vi "RRTPlan.vi"(8 "Initial Pos x,y":dbl[](array[numeric]), 9 "Dest x,y":dbl[](array[numeric]), 10 "IA State":T3={"our_robots"=[], "enemy_robots"=[], "balls"=[], "geometry"={"line_width"=0, "field_length"=0, "field_width"=0, "boundary_width"=0, "referee_width"=0, "goal_width"=0, "goal_depth"=0, "goal_wall_width"=0, "center_circle_radius"=0, "defense_radius"=0, "defense_stretch"=0, "free_kick_from_defense_dist"=0, "penalty_spot_from_field_line_dist"=0, "penalty_line_from_spot_dist"=0}, "IA Judge"={"stage"="", "command"="", "our_goalie_id"=0.0, "enemy_goalie_id"=0.0, "command enum"=enum."Halt", "Time"=enum."Azul"}, "Received Timestamp"=timestamp(0 s since 1904-01-01), "Events"={"Touch"=FALSE, "Ball out"=FALSE, "id touch"=0.0, "Ball out of \nVision"=FALSE, "Ball inside \nGoalie area"=FALSE, "Robot not responding"=FALSE, "Robots responding status"=[1.0, 1.0, 1.0, 1.0, 1.0, 1.0], "Enemy Ball \nPossession"=FALSE, "Pass State"=FALSE, "id end of pass"=0.0, "Kick"=FALSE, "Id ini Possession"=0.0, "Ball Possesion"=FALSE, "Id Possesion"=0.0}}, 11 "Robot":T4={"id"=0, "function"=enum."Attacker", "x"=0.0, "y"=0.0, "orientation"=0.0, "v_tangent"=0.0, "v_normal"=0.0, "v_ang"=0.0, "kick_x"=0.0, "kick_z"=0.0, "dribble"=FALSE, "Timestamp"=timestamp(0 s since 1904-01-01), "estimatives"={"est_v_tangent"=0.0, "est_v_normal"=0.0, "est_vx"=0.0, "est_vy"=0.0, "Pos Robot Est"=[]}, "dest_x_kick"=0.0, "dest_y_kick"=0.0, "Gap Coord"=[], "States"=enum."GoToTangent", "Path "=[], "Path  Smooth"=[], "Dest"=[]}) -> (0 "Path":dbl[][](array[numeric]), 1 "Smooth Path":dbl[][](array[numeric]))   [LabVIEW 2017]
uses:
  Core/AI Robot.ctl
  Intel/Functions Enum.ctl
  Intel/AttackerStates.ctl
  PathDests.ctl
  PathDest.ctl
  Core/AI Input.ctl
  Core/AI Ball.ctl
  Core/Field Size.ctl
  Core/AI Judge.ctl
  Intel/Command Enum.ctl
  Util/Events/Events.ctl
  kD-tree/KD-Tree.ctl
  kD-tree/Node.ctl
  <vilib>/Analysis/_algsub.llb/Real Vector Norm.vi
  <vilib>/Analysis/NI_AALPro.lvlib
panel:
  out "New KD-Tree":T1
  out "x > y? 2":bool
  out "Modulo":dbl
  in  "WayPointProb":dbl=0.6 format="%#_13g"
  in  "GoalProb":dbl=0.1 format="%#_13g"
  in  "Step":dbl=80.0
  out "Elapsed Time (s)":dbl
  out "Time has Elapsed":bool
  in  "threshold":dbl=80.0
  out "Goal":dbl[](array[numeric])
  out "Initial State":dbl[](array[numeric])
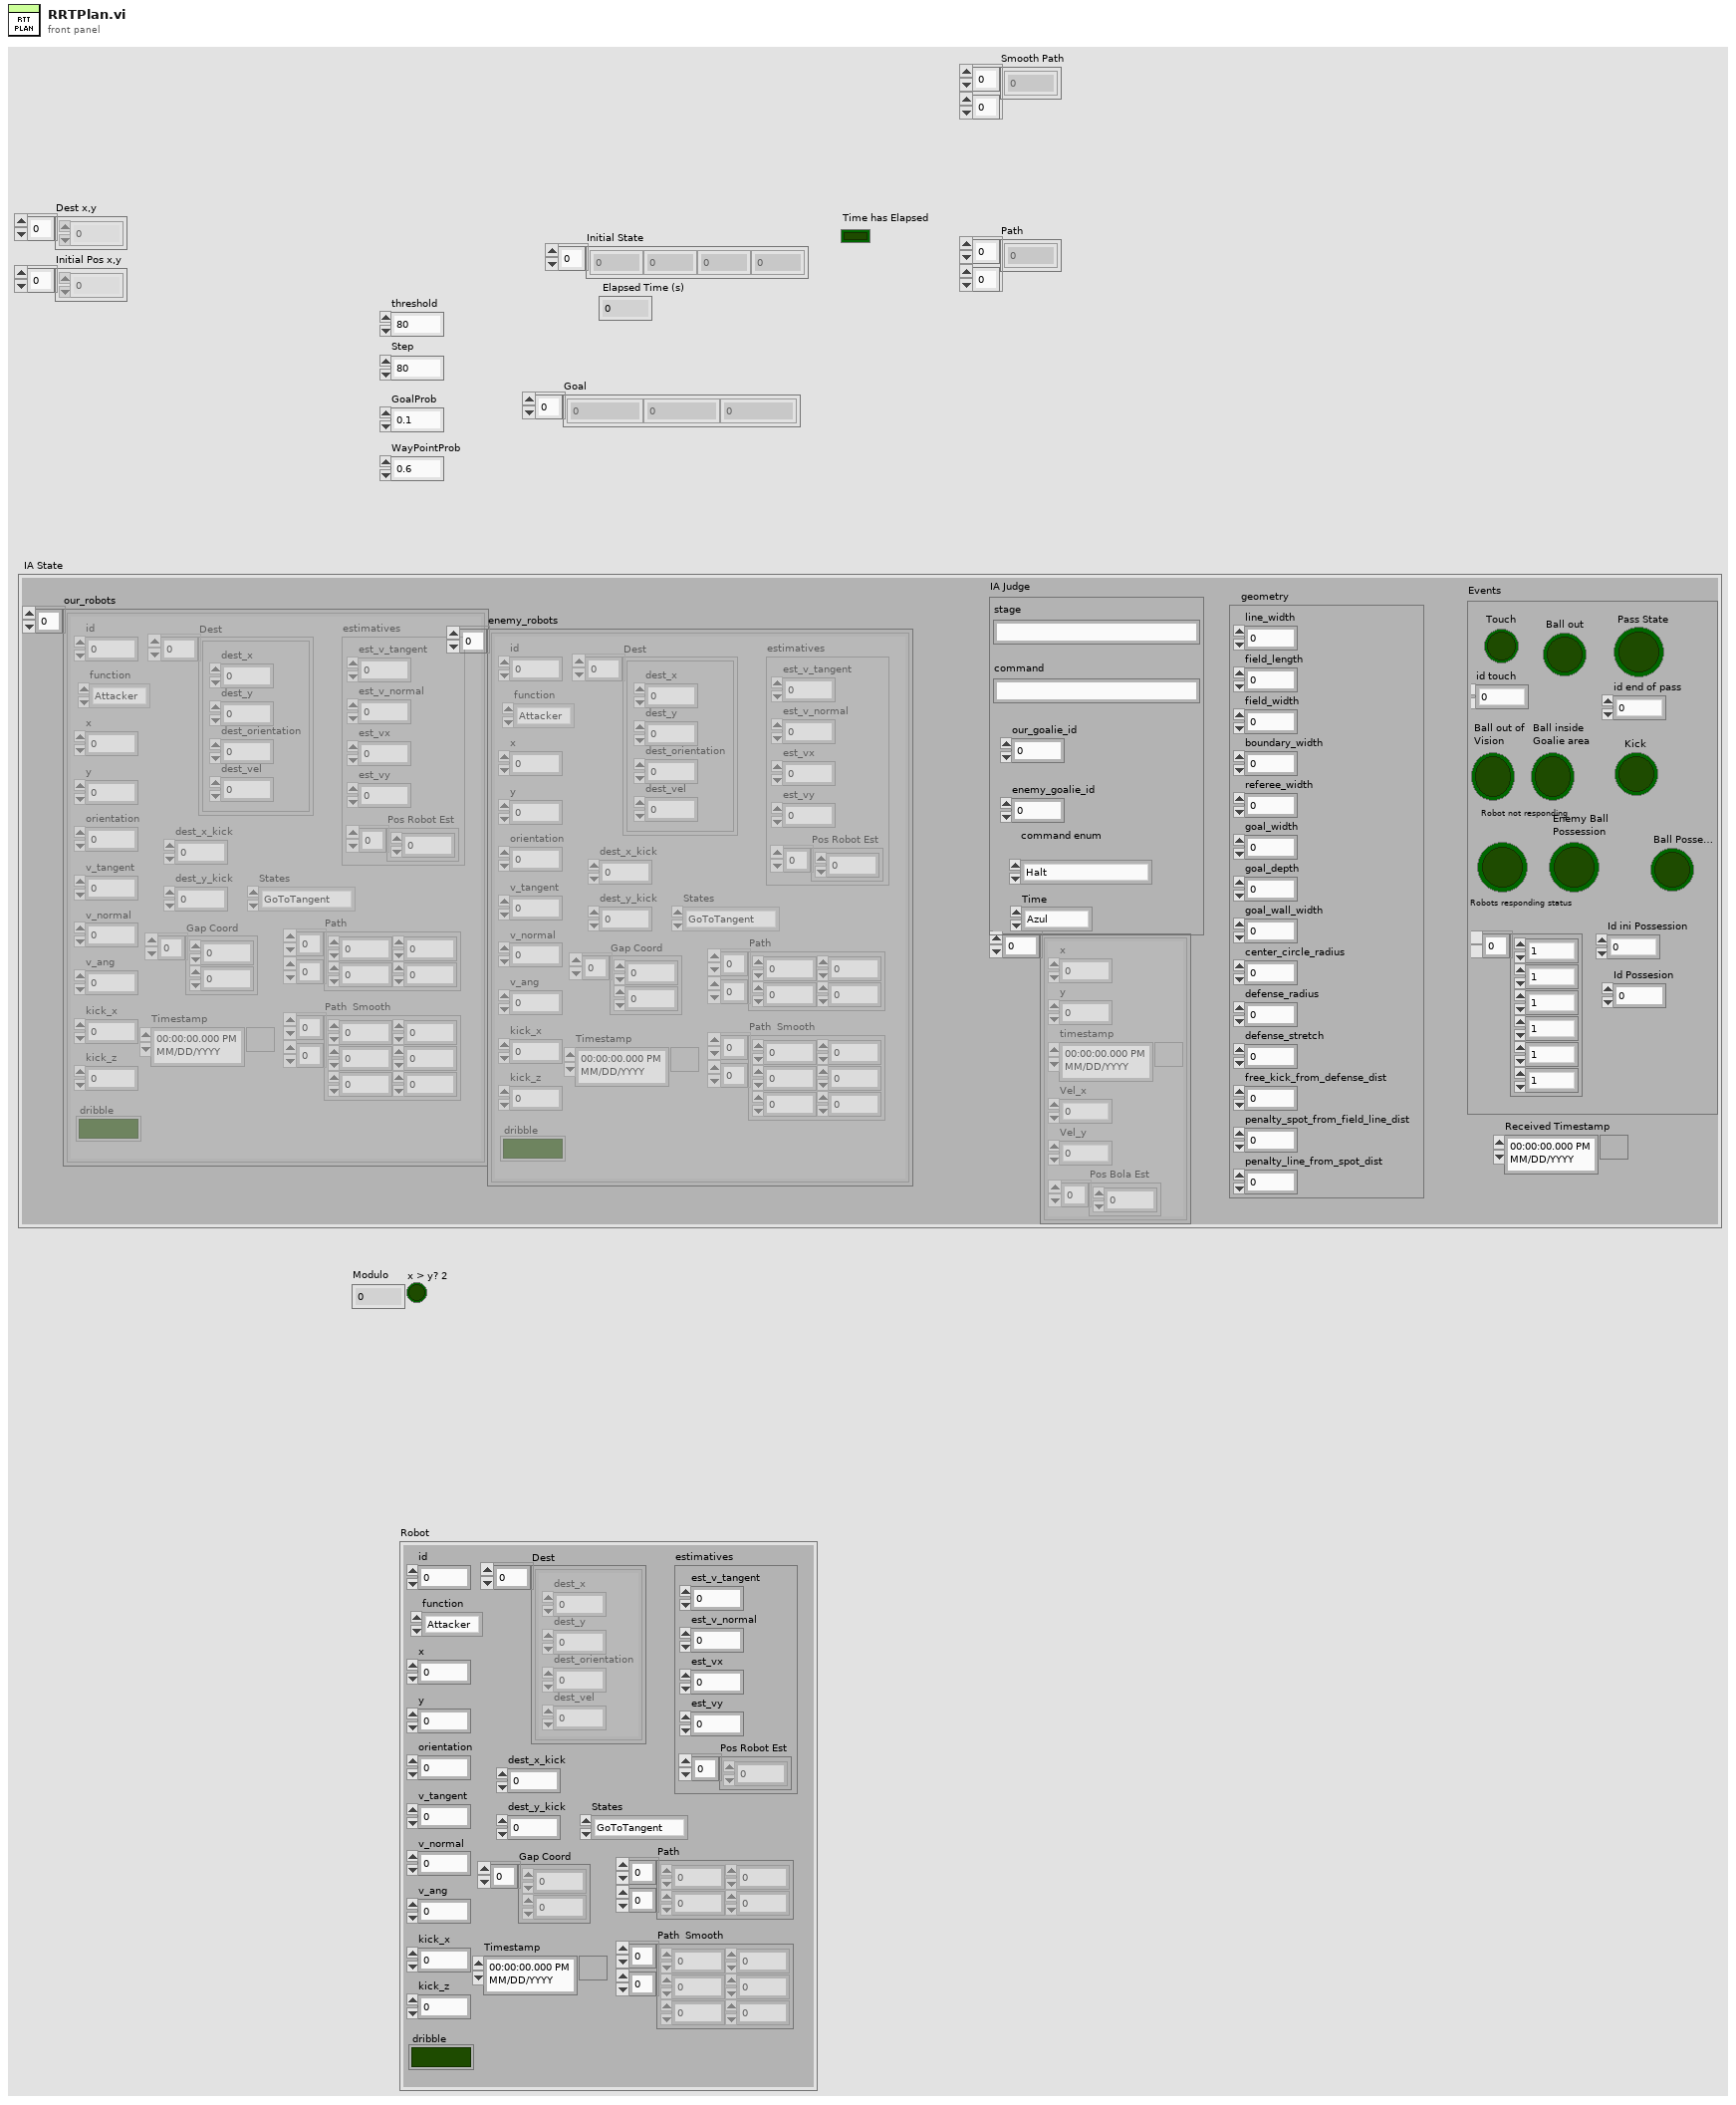
[diagram p1: front panel]
types:
  T1 = typedef "KD-Tree.ctl" = T2[]
  T2 = typedef "Node.ctl" = cluster{"axis":enum16{"null", "x", "y"}, "value":dbl, "left":dbl, "right":dbl, "Point":dbl[]}
  T3 = typedef "AI Input.ctl" = cluster{"our_robots":T4[], "enemy_robots":T4[], "balls":T9[], "geometry":T10, "IA Judge":T11, "Received Timestamp":timestamp, "Events":T13}
  T4 = typedef "AI Robot.ctl" = cluster{"id":u32, "function":T5, "x":dbl, "y":dbl, "orientation":dbl, "v_tangent":dbl, "v_normal":dbl, "v_ang":dbl, "kick_x":dbl, "kick_z":dbl, "dribble":bool, "Timestamp":timestamp, "estimatives":cluster{"est_v_tangent":dbl, "est_v_normal":dbl, "est_vx":dbl, "est_vy":dbl, "Pos Robot Est":dbl[]}, "dest_x_kick":dbl, "dest_y_kick":dbl, "Gap Coord":dbl[], "States":T6, "Path ":dbl[][], "Path  Smooth":dbl[][], "Dest":T7}
  T5 = typedef "Functions Enum.ctl" = enum16{"Attacker", "Goalie", "Defender", "Striker", "Goto 0", "Dummy", "Kicker", "ZigZag"}
  T6 = typedef "AttackerStates.ctl" = enum16{"Pass", "GoToTangent", "BallGetting", "GoToKick", ""}
  T7 = typedef "PathDests.ctl" = T8[]
  T8 = typedef "PathDest.ctl" = cluster{"dest_x":dbl, "dest_y":dbl, "dest_orientation":dbl, "dest_vel":dbl}
  T9 = typedef "AI Ball.ctl" = cluster{"x":dbl, "y":dbl, "timestamp":timestamp, "Vel_x":dbl, "Vel_y":dbl, "Pos Bola Est":dbl[]}
  T10 = typedef "Field Size.ctl" = cluster{"line_width":u32, "field_length":u32, "field_width":u32, "boundary_width":u32, "referee_width":u32, "goal_width":u32, "goal_depth":u32, "goal_wall_width":u32, "center_circle_radius":u32, "defense_radius":u32, "defense_stretch":u32, "free_kick_from_defense_dist":u32, "penalty_spot_from_field_line_dist":u32, "penalty_line_from_spot_dist":u32}
  T11 = typedef "AI Judge.ctl" = cluster{"stage":string, "command":string, "our_goalie_id":dbl, "enemy_goalie_id":dbl, "command enum":T12, "Time":enum16{"Azul", "Amarelo"}}
  T12 = typedef "Command Enum.ctl" = enum16{"Halt", "Stop", "Force Start", "PKA Normal Start", "Prepare Kickoff Ally", "PKE Normal Start", "Prepare Kickoff Enemy", "Prepare Penalty Ally", "PPA Normal Start", "Prepare Penalty Enemy", "PPE Normal Start", "Direct Free Enemy", "Direct Free Ally", "Indirect Free Enemy", "Indirect Free Ally", "Timeout Enemy", "Timeout Ally", "Goal Enemy", "Goal Ally", "Ball Placement Enemy", "Ball Placement Ally", "Normal Half Time", "Extra Time Break", "Extra Half Time", "None", "Post Game"}
  T13 = typedef "Events.ctl" = cluster{"Touch":bool, "Ball out":bool, "id touch":dbl, "Ball out of \nVision":bool, "Ball inside \nGoalie area":bool, "Robot not responding":bool, "Robots responding status":dbl[], "Enemy Ball \nPossession":bool, "Pass State":bool, "id end of pass":dbl, "Kick":bool, "Id ini Possession":dbl, "Ball Possesion":bool, "Id Possesion":dbl}
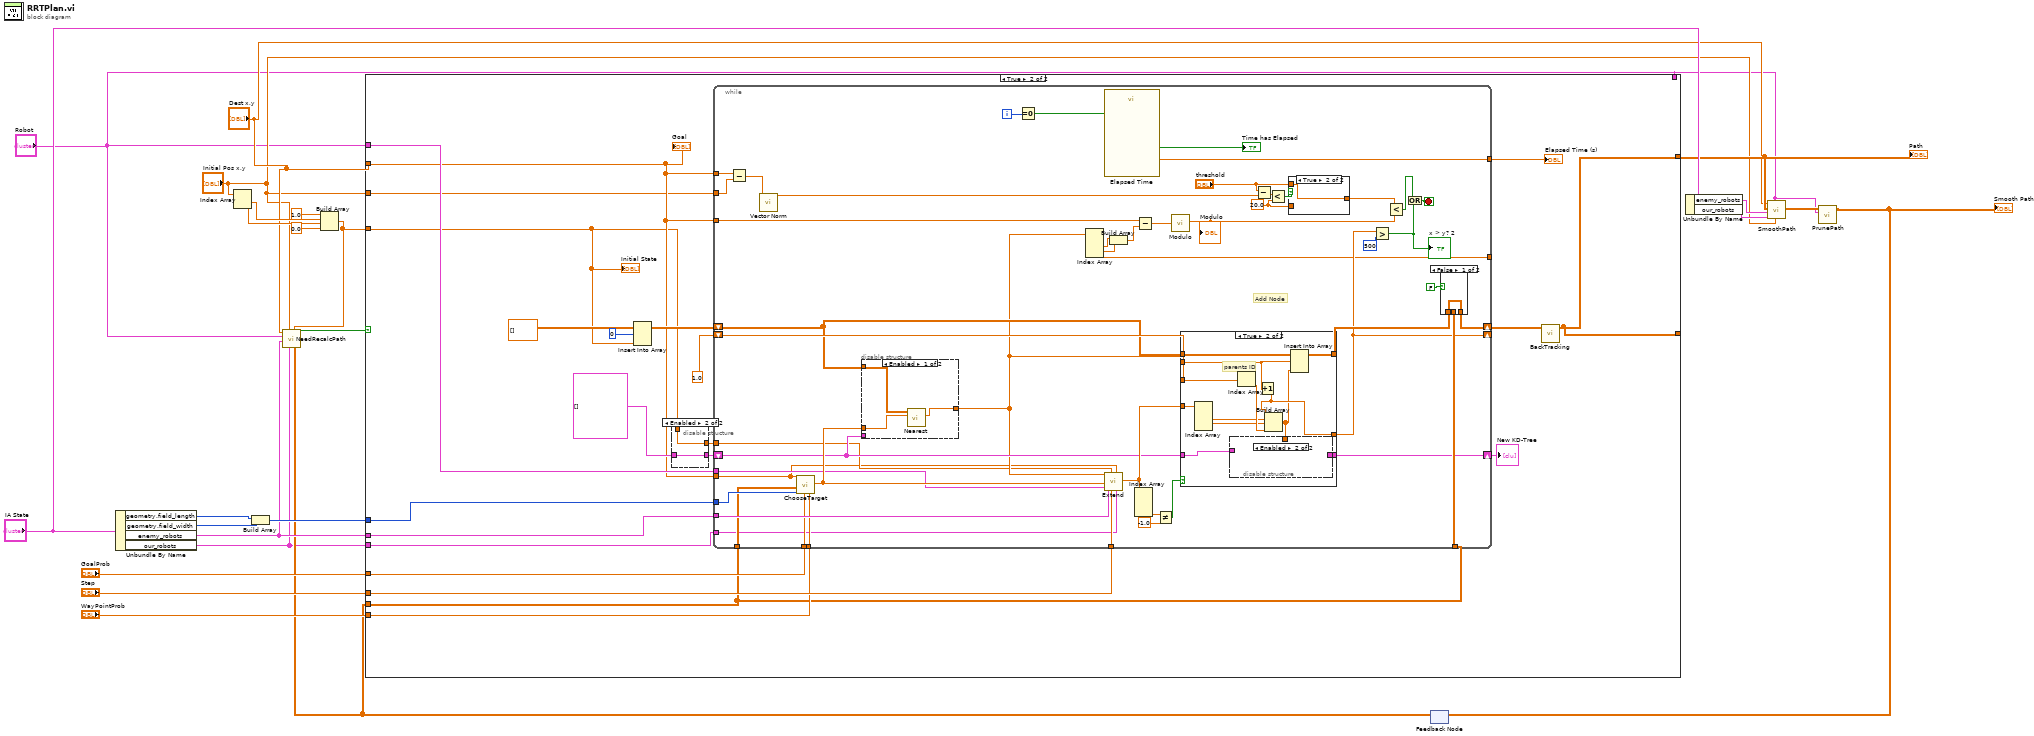
[diagram p0: block diagram]
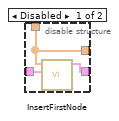
[diagram p3: hidden frame]
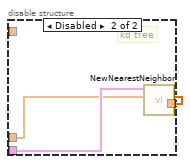
[diagram p4: hidden frame]
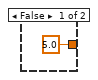
[diagram p5: hidden frame]
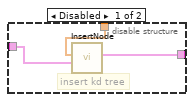
[diagram p8: hidden frame]
diagram:
  n1 = Unbundle By Name("IA State") -> ("geometry.field_length"=w24:u32, "geometry.field_width"=w23:u32, "enemy_robots"=w18:T4[], "our_robots"=w12:T4[])
  n2 = Index Array(array="Initial Pos x,y") -> (element #1=w11:dbl, element #2=w10:dbl)  [unwired: 2 in]
  n3 = Build Array(w24, w23) -> (w22:u32[])
  n4 = Build Array(1.0 ("element"), w11, w10, 0.0 ("element")) -> (w15:dbl[])
  n5 = feedback #1() -> (w14:dbl[][])  [unwired: 1 in]
  n6 = call "NeedRecalcPath.vi"("SmoothPath"=w14, "Initial State"=w15, "our_robots"=w12, "Pos x,y"="Initial Pos x,y", "enemy_robots"=w18, "Robot"="Robot", "Dest x,y"="Dest x,y") -> ("Boolean"=w13:bool)  [unwired: 4 in]
  n7 = case shown="True" w13 {
    tunnel: w22 -> [_ w37]
    tunnel: "Step" -> [_ w44]
    tunnel: "Robot" -> [_ w32]
    tunnel: "GoalProb" -> [_ w42]
    tunnel: "WayPointProb" -> [_ w41]
    tunnel: w18 -> [_ w40]
    tunnel: w14 -> [w25 w39]
    tunnel: [w25 w30] -> w6
    tunnel: "Robot" -> [_ _]
    tunnel: [w25 w30] -> _
    tunnel: "Dest x,y" -> [_ w29]
    tunnel: "Initial Pos x,y" -> [_ w28]
    tunnel: w15 -> [_ w27]
    tunnel: w12 -> [_ w26]
    frame False {
    }
    frame True {
      n8 = Insert Into Array(array=dbl[][] [] ("Pontos"), index (row)=0, new element=w27) -> (w45:dbl[][])  [unwired: 1 in]
      n9 = disable-structure shown="Enabled" {
        disable-tunnel: [w50 w52] -> w35
        disable-tunnel: T1 [] ("New KD-Tree") -> [w49 w52]
        disable-tunnel: w27 -> [w48 w51]
        disable-tunnel: [w48 w51] -> w31
        frame Disabled {
          n10 = call "InsertFirstNode.vi"("New KD-Tree in"=w49, "Tree"=w48) -> ("New KD-Tree out"=w50:T1)  [unwired: 9 in]
        }
        frame Enabled {
        }
      }
      n11 = while {
        tunnel: w29 -> [w100]
        tunnel: w29 -> [w55]
        tunnel: w37 -> [w97]
        shift-right: [w81] -> w38
        shift-left: w45 -> [w80]
        tunnel: w40 -> [w95]
        tunnel: w44 -> [w94]
        shift-right: [w77] -> _
        shift-left: 1.0 -> [w85]
        tunnel: w39 -> [w84]
        tunnel: w39 -> [w83]
        tunnel: w42 -> [w75]
        tunnel: w41 -> [w74]
        tunnel: [w71] -> _
        tunnel: w29 -> [w70]
        shift-right: [w63] -> w36
        shift-left: w35 -> [w62]
        tunnel: [w60] -> w33
        tunnel: w32 -> [w57]
        tunnel: w31 -> [w56]
        tunnel: w28 -> [w54]
        tunnel: w26 -> [w53]
        i -> [w59]
        stop <- w89 stop-if-true
        w64 = 20.0 ("y")
        # "Add Node"
        n12 = Subtract(x=w70, y=w54) -> (x-y=w69:dbl[])
        n13 = call-poly <vilib>:"Vector Norm.vi"("Input Vector"=w69) -> ("norm"=w67:dbl)  [unwired: 9 in, 1 out]
        n14 = call "ChooseTarget.vi"("WayPointProb"=w74, "GoalProb"=w75, "Field Geometry"=w97, "WayPointCache"=w84, "Goal"=w55) -> ("Target"=w96:dbl[])  [unwired: 6 in]
        n15 = disable-structure shown="Enabled" {
          disable-tunnel: w96 -> [w104 w106]
          disable-tunnel: w80 -> [w103 _]
          disable-tunnel: w62 -> [_ w107]
          disable-tunnel: [w102 w105] -> w61
          frame Enabled {
            n16 = call "Nearest.vi"("Target"=w104, "Pontos"=w103) -> ("Nearest"=w102:dbl[])  [unwired: 9 in]
          }
          frame Disabled {
            # "kd tree"
            n17 = call "NewNearestNeighbor.vi"("q"=w106, "KD-Tree"=w107) -> ("Nearest"=w105:dbl[])  [unwired: 9 in]
          }
        }
        n18 = Equal To 0?(x=w59) -> (x = 0?=w58:bool)
        n19 = Index Array(array=w61) -> (element #2=w88:dbl, element #3=w87:dbl, element #4=w71:dbl)  [unwired: 4 in, 1 out]
        n20 = call "Elapsed Time"("Auto Reset"=w58) -> ("Elapsed Time (s)"=w60:dbl, "Time has Elapsed"=→"Time has Elapsed":bool)  [unwired: 11 in, 6 out]
        n21 = call "Extend.vi"("our_robots"=w53, "Goal"=w55, "Step"=w94, "Initial State"=w56, "enemy_robots"=w95, "Robot in"=w57, "Target"=w96, "Nearest"=w61) -> ("New State"=w90:dbl[])  [unwired: 3 in]
        n22 = Build Array(w88, w87) -> (w86:dbl[])
        n23 = Index Array(array=w90) -> (element #4=w93:dbl)  [unwired: 4 in, 3 out]
        n24 = Subtract(x=w100, y=w86) -> (x-y=w101:dbl[])
        n25 = Not Equal?(x=w93, y=-1.0) -> (x != y?=w91:bool)
        n26 = call "Modulo.vi"("2D vector"=w101) -> ("Modulo"=w99:dbl)  [unwired: 10 in]
        "Modulo" <- w99
        n27 = case shown="True" w91 {
          tunnel: w80 -> [w114 w126]
          tunnel: [w114 w122] -> w82
          tunnel: w90 -> [_ w125]
          tunnel: w85 -> [w113 w121]
          tunnel: w61 -> [_ w124]
          tunnel: [w113 w116] -> w77
          tunnel: [w112 w120] -> w63
          tunnel: w62 -> [w112 w119]
          frame False {
          }
          frame True {
            # "parents ID"
            n28 = Index Array(array=w125) -> (element #2=w118:dbl, element #3=w117:dbl)  [unwired: 4 in, 2 out]
            n29 = Index Array(array=w124) -> (element=w123:dbl)  [unwired: 1 in]
            n30 = Increment(x=w121) -> (x+1=w116:dbl)
            n31 = Build Array(w116, w118, w117, w123) -> (w115:dbl[])
            n32 = disable-structure shown="Enabled" {
              disable-tunnel: [w129 _] -> w120
              disable-tunnel: w119 -> [w128 _]
              disable-tunnel: w115 -> [w127 _]
              frame Disabled {
                # "insert kd tree"
                n33 = call "InsertNode.vi"("KD-Tree"=w128, "New Node"=w127) -> ("New KD-Tree"=w129:T1)  [unwired: 9 in]
              }
              frame Enabled {
              }
            }
            n34 = Insert Into Array(array=w126, index (row)=w121, new element=w115) -> (w122:dbl[][])  [unwired: 1 in]
          }
        }
        n35 = Subtract(x="threshold", y=w67) -> (x-y=w65:dbl)
        n36 = Less?(x=w65, y=w64) -> (x < y?=w66:bool)
        n37 = case shown="True" w66 {
          tunnel: [5.0 ("threshold") w109] -> w98
          tunnel: "threshold" -> [_ w109]
          tunnel: w64 -> [_ _]
          frame False {
          }
          frame True {
          }
        }
        n38 = Greater?(x=w77, y=500) -> (0:w72:bool)
        "x > y? 2" <- w72
        n39 = Less?(x=w99, y=w98) -> (x < y?=w73:bool)
        n40 = Or(x=w73, y=w72) -> (x .or. y?=w89:bool)
        n41 = case shown="False" FALSE {
          tunnel: w83 -> [_ w111]
          tunnel: [w110 w111] -> w81
          tunnel: w82 -> [w110 _]
          frame False {
          }
          frame True {
          }
        }
      }
      "New KD-Tree" <- w36
      "Elapsed Time (s)" <- w33
      n42 = call "BackTracking.vi"("Pontos"=w38) -> ("Path"=w30:dbl[][])  [unwired: 9 in, 1 out]
      "Initial State" <- w27
      "Goal" <- w29
    }
  }
  "Path" <- w6
  n43 = Unbundle By Name("IA State") -> ("enemy_robots"=w7:T4[], "our_robots"=w8:T4[])
  n44 = call "SmoothPath.vi"("Initial State"="Initial Pos x,y", "Robot in"="Robot", "our_robots"=w8, "enemy_robots"=w7, "Path"=w6, "Goal"="Dest x,y") -> ("SmoothPath"=w3:dbl[][])  [unwired: 5 in]
  n45 = call "PrunePath.vi"("Robot in"="Robot", "Path in"=w3) -> ("Path out"=w2:dbl[][])  [unwired: 8 in, 1 out]
  "Smooth Path" <- w2
  n46 = feedback-in #1(w2) -> ()
